vi "Graph with cursors Test.vi"() -> ()   [LabVIEW 2014, in "Graph with cursors XControl.xctl"]
uses:
  Graph with cursors XControl.xctl
  <vilib>/measure/NI_MABase.lvlib
panel:
  in  "stop":bool
  out "Graph with cursors XControl":waveform(dbl)(xcontrol)
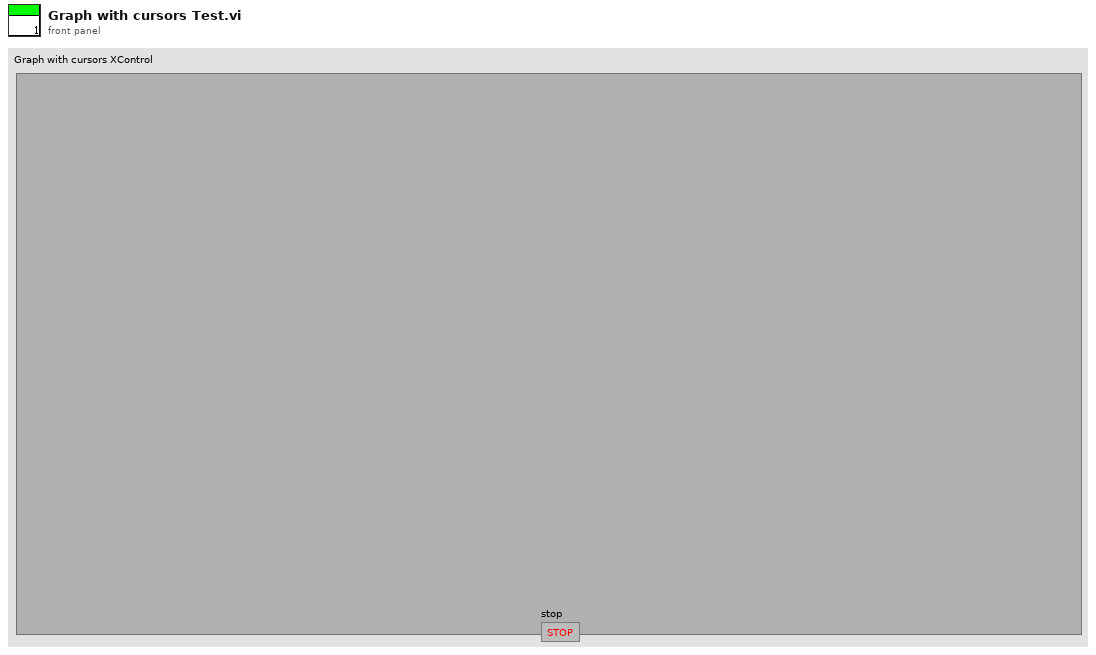
[diagram p1: front panel]
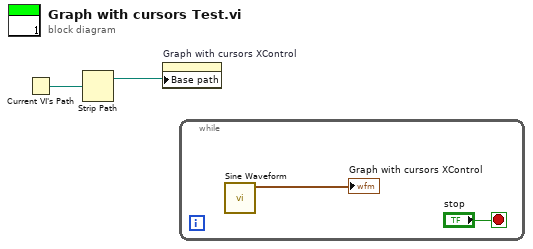
[diagram p0: block diagram]
diagram:
  n1 = Current VI's Path() -> (path=w2:path)
  n2 = Strip Path(path=w2) -> (stripped path=w1:path)  [unwired: 1 out]
  n3 = property on="Graph with cursors XControl" class="Graph with cursors XControl (st"("Base path"=w1) -> ()  [unwired: 2 in, 2 out]
  n4 = while {
    stop <- "stop" stop-if-true
    n5 = call <vilib>:"Sine Waveform.vi"() -> ("signal out"=→"Graph with cursors XControl":waveform(dbl))  [unwired: 10 in, 1 out]
  }
